vi "Analyze Fan Acceleration (FPGA).vi"(10 "max acceleration threshold (g)":sgl, 11 "acceleration (g)":sgl) -> (3 "max acceleration exceeded?":bool)   [LabVIEW 2017]
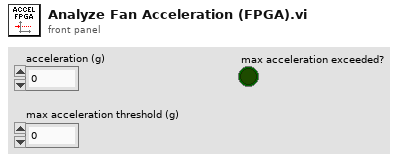
[diagram p1: front panel]
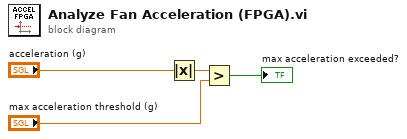
[diagram p0: block diagram]
diagram:
  n1 = Absolute Value(x="acceleration (g)") -> (abs(x)=w4:sgl)
  n2 = Greater?(x=w4, y="max acceleration threshold (g)") -> (0:→"max acceleration exceeded?":bool)
